vi "dvp Vi Get Flip Vertical State.vi"(10 "pFlipVerticalState":i32, 11 "handle":u32) -> (2 "pFlipVerticalState out":i32, 3 "function return":u32(ring))   [LabVIEW 2018, in "LabViewDVPCamera.lvlib"]
doc: "LabviewDvp2Api dvpStatus dvpViGetFlipVerticalState(dvpHandle handle, BOOL *pFlipVerticalState);"
uses:
  LabViewDVPCamera.lvlib
  LabViewDVPCamera/LabViewDVPCamera.dll
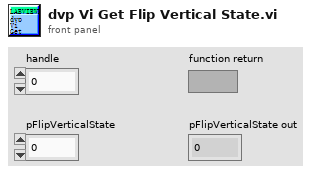
[diagram p1: front panel]
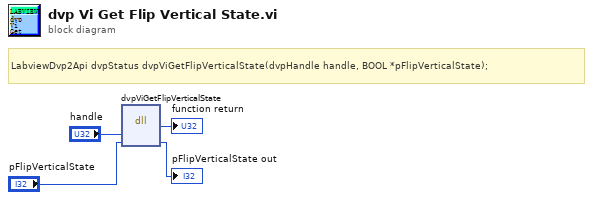
[diagram p0: block diagram]
diagram:
  # "LabviewDvp2Api dvpStatus dvpViGetFlipVerticalState(dvpHandle handle, BOOL *pFlipVerticalState);"
  n1 = dll-call lib="C:/Program Files (x86)/DVP2 Labview cn 64/Sample/LabViewDVPCamera/LabViewDVPCamera.*" fn="dvpViGetFlipVerticalState"("handle"="handle", "pFlipVerticalState"="pFlipVerticalState") -> (→"function return":u32, "pFlipVerticalState"=→"pFlipVerticalState out":i32)  [unwired: 4 in, 2 out]
